vi "Write License Text to VI Description.vi"(8 "error in (no error)":errorcluster, 10 "String":string, 11 "VI in":refnum<vi>) -> (0 "error out":errorcluster, 3 "VI out":refnum<vi>)   [LabVIEW 2012, in "Add License to VI Documentation.lvlib"]
uses:
  Add License to VI Documentation.lvlib
  <vilib>/Utility/error.llb/whitespace.ctl
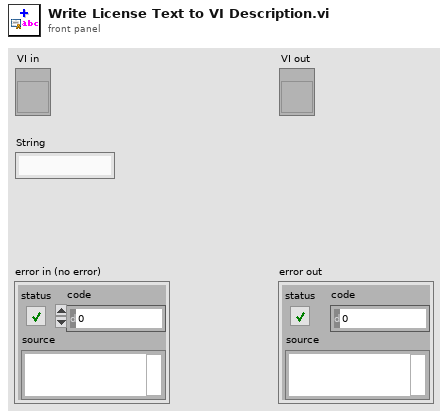
[diagram p1: front panel]
types:
  T1 = typedef "whitespace.ctl" = u16
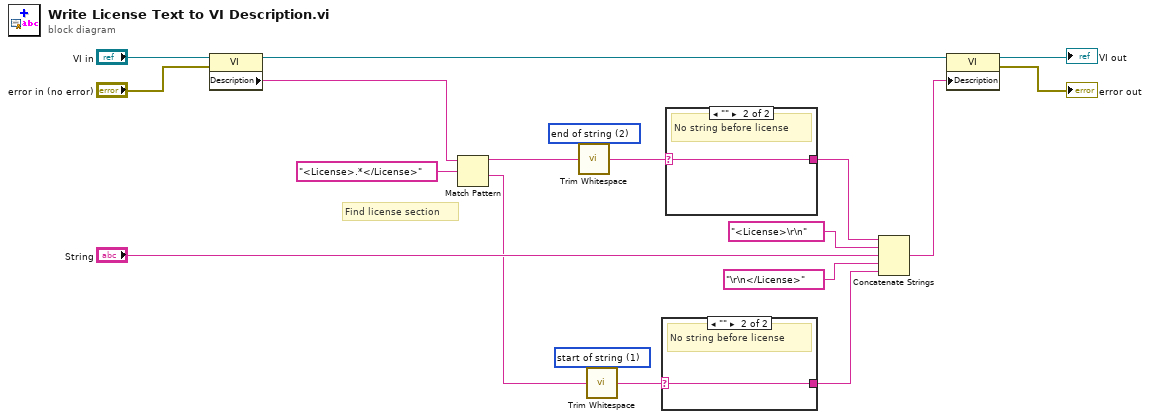
[diagram p0: block diagram]
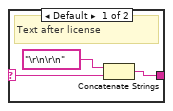
[diagram p2: hidden frame]
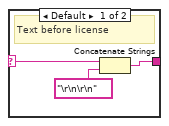
[diagram p3: hidden frame]
diagram:
  w5 = T1 1 items=["both", "start of string", "end of string"] ("location (both)")
  w6 = T1 2 items=["both", "start of string", "end of string"] ("location (both)")
  # "Find license section"
  n1 = property on="Property Node" class="VI"(reference="VI in", error in="error in (no error)") -> (reference out=w16:refnum<vi>, "Description"=w12:string)  [unwired: 1 out]
  n2 = Match Pattern(string=w12, regular expression="<License>.*</License>") -> (before substring=w8:string, after substring=w7:string)  [unwired: 1 in, 2 out]
  n3 = call <vilib>:"Trim Whitespace.vi"("string"=w8, "location (both)"=w6) -> ("trimmed string"=w4:string)
  n4 = call <vilib>:"Trim Whitespace.vi"("string"=w7, "location (both)"=w5) -> ("trimmed string"=w2:string)
  n5 = case shown="\"\"" w2 {
    selector: w2 -> [w22 w23]
    tunnel: [w20 w23] -> w1
    frame Default {
      # "Text after license"
      n6 = Concatenate Strings("\r\n\r\n" ("string"), w22) -> (w20:string)
    }
    frame "" {
      # "No string before license"
    }
  }
  n7 = case shown="\"\"" w4 {
    selector: w4 -> [w26 w27]
    tunnel: [w24 w27] -> w3
    frame Default {
      # "Text before license"
      n8 = Concatenate Strings(w26, "\r\n\r\n" ("string")) -> (w24:string)
    }
    frame "" {
      # "No string before license"
    }
  }
  n9 = Concatenate Strings(w3, "<License>\r\n" ("string"), "String", "\r\n</License>" ("string"), w1) -> (w17:string)
  n10 = property on="Property Node" class="VI"(reference=w16, "Description"=w17) -> (reference out=→"VI out":refnum<vi>, error out=→"error out":errorcluster)  [unwired: 1 in]
